vi "Circular Buffer (scaler).vi"(6 "History Length [1024]":i32=1024, 7 "reset":bool, 8 "error in":errorcluster, 11 "Element in":dbl) -> (0 "error out":errorcluster, 3 "Array out":dbl[](array[numeric]))   [LabVIEW 2019, in "xy_utilities.lvlib"]
doc: "Circular Buffer with controllable reset and history length."
uses:
  xy_utilities.lvlib
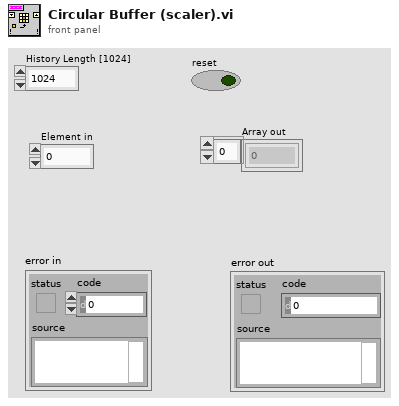
[diagram p1: front panel]
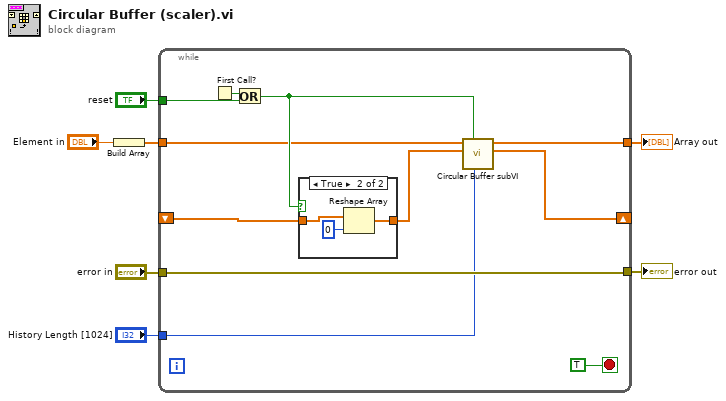
[diagram p0: block diagram]
diagram:
  n1 = Build Array("Element in") -> (w1:dbl[])
  n2 = while {
    tunnel: w1 -> [w8]
    tunnel: [w18] -> w7
    tunnel: "error in" -> [w18]
    tunnel: "reset" -> [w16]
    shift-right: [w12] -> _
    shift-left: _ -> [w10]
    tunnel: [w13] -> w4
    tunnel: "History Length [1024]" -> [w14]
    stop <- TRUE stop-if-true
    n3 = First Call?() -> (First Call?: T/F=w17:bool)
    n4 = Or(x=w17, y=w16) -> (x .or. y?=w11:bool)
    n5 = case shown="True" w11 {
      tunnel: w10 -> [w19 w20]
      tunnel: [w19 w21] -> w9
      frame False {
      }
      frame True {
        n6 = Reshape Array(w20, 0 ("dimension size")) -> (w21:dbl[])
      }
    }
    n7 = call "Circular Buffer subVI.vi"("History Length [1024]"=w14, "Reset"=w11, "Buffer in"=w9, "Array in"=w8) -> ("Buffer out"=w12:dbl[], "Array out"=w13:dbl[])  [unwired: 6 in]
  }
  "Array out" <- w4
  "error out" <- w7
